vi "Simulate GPS Coordinates.vi"(0 "Previous Latitude":dbl, 1 "Previous Longitude":dbl, 2 "Drive Voltage":dbl=1.0, 3 "Destination Latitude":dbl format="%#_11g", 4 "Destination Longitude":dbl format="%#_11g") -> (5 "Current Latitude":dbl format="%#_8g", 6 "Current Longitude":dbl format="%#_9g")   [LabVIEW 2011]
panel:
  out "Longitude Difference":dbl
  out "Latitude Difference":dbl
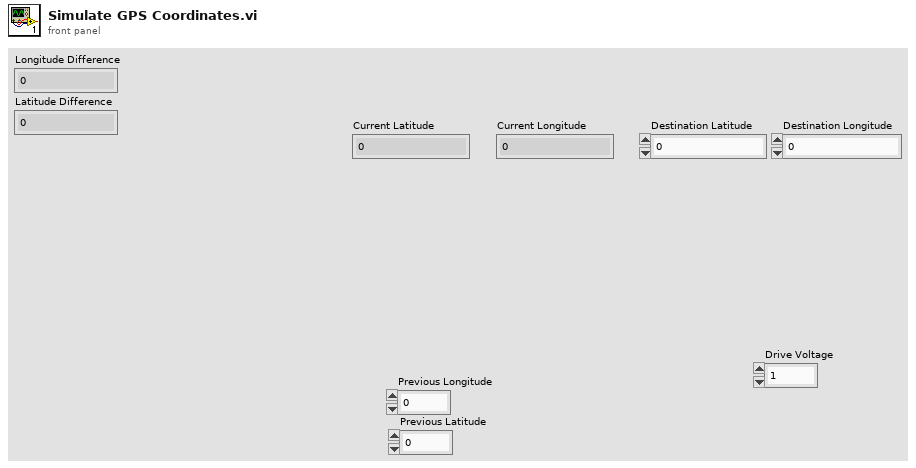
[diagram p1: front panel]
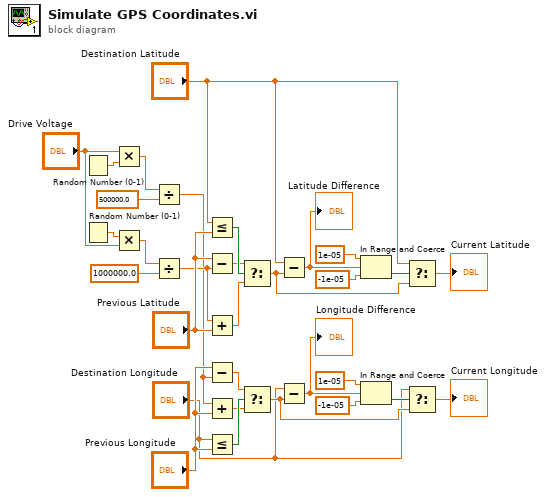
[diagram p0: block diagram]
diagram:
  n1 = Random Number (0-1)() -> (number: 0 to 1=w11:dbl)
  n2 = Random Number (0-1)() -> (number: 0 to 1=w9:dbl)
  n3 = Multiply(x="Drive Voltage", y=w11) -> (x*y=w10:dbl)
  n4 = Multiply(x=w9, y="Drive Voltage") -> (x*y=w8:dbl)
  n5 = Divide(x=w10, y=500000.0) -> (x/y=w18:dbl)
  n6 = Divide(x=w8, y=1000000.0) -> (x/y=w19:dbl)
  n7 = Less Or Equal?(x="Destination Latitude", y="Previous Latitude") -> (x <= y?=w22:bool)
  n8 = Subtract(x="Previous Latitude", y=w19) -> (x-y=w20:dbl)
  n9 = Add(x=w19, y="Previous Latitude") -> (x+y=w21:dbl)
  n10 = Subtract(x="Previous Longitude", y=w18) -> (x-y=w17:dbl)
  n11 = Add(x=w18, y="Previous Longitude") -> (x+y=w16:dbl)
  n12 = Less Or Equal?(x="Destination Longitude", y="Previous Longitude") -> (x <= y?=w23:bool)
  n13 = Select(t=w20, s=w22, f=w21) -> (s? t:f=w15:dbl)
  n14 = Select(t=w17, s=w23, f=w16) -> (s? t:f=w13:dbl)
  n15 = Subtract(x="Destination Latitude", y=w15) -> (x-y=w14:dbl)
  "Latitude Difference" <- w14
  n16 = Subtract(x="Destination Longitude", y=w13) -> (x-y=w12:dbl)
  "Longitude Difference" <- w12
  n17 = In Range and Coerce(upper limit=1e-05, x=w14, lower limit=-1e-05) -> (In Range?=w27:bool)  [unwired: 1 out]
  n18 = In Range and Coerce(upper limit=1e-05, x=w12, lower limit=-1e-05) -> (In Range?=w24:bool)  [unwired: 1 out]
  n19 = Select(t="Destination Latitude", s=w27, f=w15) -> (s? t:f=→"Current Latitude":dbl)
  n20 = Select(t="Destination Longitude", s=w24, f=w13) -> (s? t:f=→"Current Longitude":dbl)
